vi "GV preframeclock.vi"() -> ()   [LabVIEW 2017]
panel:
  out "Preframeclock":bool
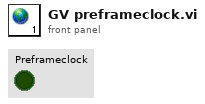
[diagram p1: front panel]
diagram:
